vi "Toggle.vi"(1 "Input":bool) -> (0 "Output":bool)   [LabVIEW 2013]
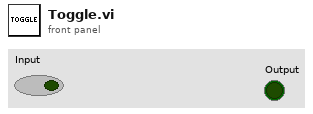
[diagram p1: front panel]
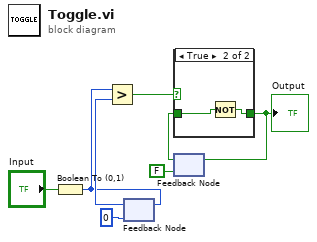
[diagram p0: block diagram]
diagram:
  n1 = Boolean To (0,1)(Boolean="Input") -> (0, 1=w5:i16)
  n2 = feedback #1(i16 0) -> (w6:i16)
  n3 = Greater?(x=w5, y=w6) -> (0:w4:bool)
  n4 = feedback-in #1(w5) -> ()
  n5 = feedback #2(FALSE) -> (w2:bool)
  n6 = case shown="True" w4 {
    tunnel: [w9 w11] -> w3
    tunnel: w2 -> [w9 w10]
    frame False {
    }
    frame True {
      n7 = Not(x=w10) -> (.not. x?=w11:bool)
    }
  }
  "Output" <- w3
  n8 = feedback-in #2(w3) -> ()
